vi "R1DOControl_SetParams.vi"(7 "LabVIEW Web Service Request":refnum<class "Web Request.lvclass">, 8 "N2ValveGain":dbl, 9 "AirValveGain":dbl, 10 "Tolerance":dbl, 11 "SetPoint":dbl) -> (2 "ControlStatus":string, 3 "DO_SetParams_out":T1)   [LabVIEW 2016]
uses:
  <vilib>/wsapi/Web Request.lvclass
panel:
  # "Use the Web Service Request input terminal to call the VIs on the Web Services palette. Do not remove it from the connector pane unless you don't need access to the palette."
  # "Each additional control wired to the connector pane will be available as an input in the URL. To include an indicator in terminal-mode output (the default setting), it must also be wired to the connector pane."
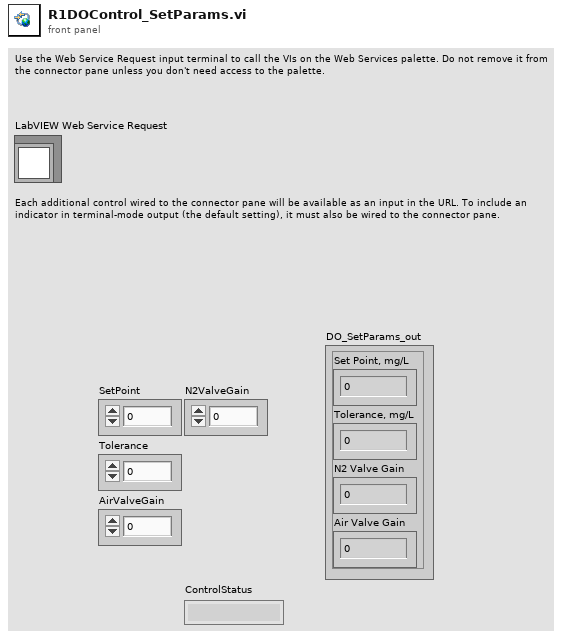
[diagram p1: front panel]
types:
  T1 = cluster{"Set Point, mg/L":dbl, "Tolerance, mg/L":dbl, "N2 Valve Gain":dbl, "Air Valve Gain":dbl}
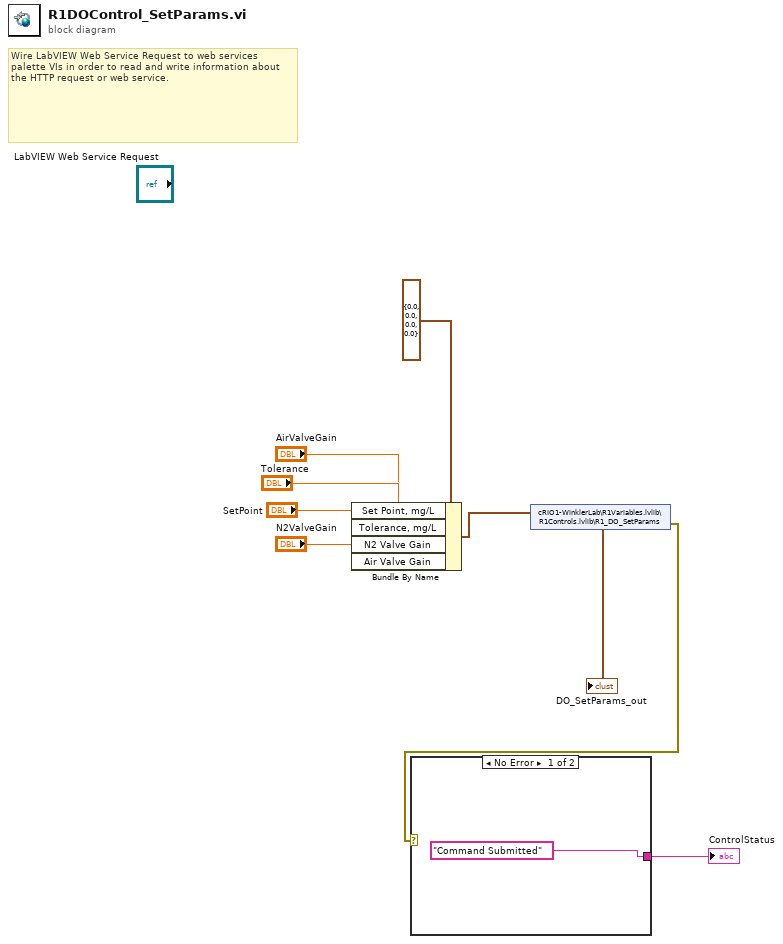
[diagram p0: block diagram]
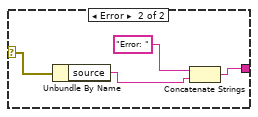
[diagram p2: hidden frame]
diagram:
  # "Wire LabVIEW Web Service Request to web services palette VIs in order to read and write information about the HTTP request or web service."
  n1 = Bundle By Name(cluster=T1 {"Set Point, mg/L"=0.0, "Tolerance, mg/L"=0.0, "N2 Valve Gain"=0.0, "Air Valve Gain"=0.0} ("R1_DO_SetParams"), "Set Point, mg/L"="SetPoint", "Tolerance, mg/L"="Tolerance", "N2 Valve Gain"="N2ValveGain", "Air Valve Gain"="AirValveGain") -> (w7:T1)
  "DO_SetParams_out" <- w7
  n2 = shared-variable "cRIO1-WinklerLab\\R1Variables.lvlib\\R1Controls.lvlib\\R1_DO_SetParams"(w7) -> (error out=w2:errorcluster)  [unwired: 1 in]
  n3 = case shown="No Error" w2 {
    selector: w2 -> [_ w11]
    tunnel: ["Command Submitted" ("ControlStatus") w10] -> w1
    frame No Error {
    }
    frame Error {
      n4 = Unbundle By Name(w11) -> ("source"=w12:string)
      n5 = Concatenate Strings("Error: ", w12) -> (w10:string)
    }
  }
  "ControlStatus" <- w1
